vi "Handshake.vi"(8 "error in (no error)":errorcluster, 11 "Connection.NetworkStream":refnum<class "Connection.NetworkStream.lvclass">) -> (0 "error out":errorcluster, 3 "Connection.NetworkStream":refnum<class "Connection.NetworkStream.lvclass">)   [LabVIEW 2013]
uses:
  Connection.NetworkStream/Connection.NetworkStream.lvclass
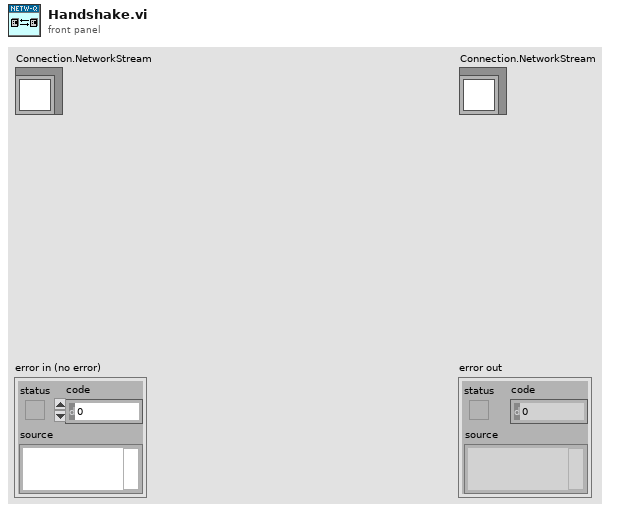
[diagram p1: front panel]
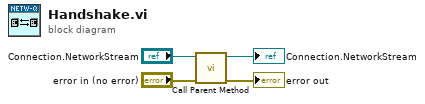
[diagram p0: block diagram]
diagram:
  n1 = call-parent "Call Parent Method"("error in (no error)"="error in (no error)", "Connection in"="Connection.NetworkStream") -> ("error out"=→"error out":errorcluster, "Connection out"=→"Connection.NetworkStream":refnum<class "Connection.NetworkStream.lvclass">)  [unwired: 8 in]
